vi "H5Pget_alloc_time.vi"(6 "error in (no error)":errorcluster, 9 "HDF5 Property Ref":T2) -> (0 "error out":errorcluster, 2 "Alloc Time":T1 items=["H5D_ALLOC_TIME_ERROR"=-1, "H5D_ALLOC_TIME_DEFAULT"=0, "H5D_ALLOC_TIME_EARLY"=1, "H5D_ALLOC_TIME_LATE"=2, "H5D_ALLOC_TIME_INCR"=3], 3 "HDF5 Ref out":T2)   [LabVIEW 2017]
doc: "Retrieves the timing for storage space allocation."
uses:
  <vilib>/UPVI/lvhdf5/library.llb/HDF5 Ref.ctl
  <vilib>/UPVI/lvhdf5/property.llb/H5D_alloc_time_t.ctl
  <vilib>/UPVI/lvhdf5/hdf5.dll
panel:
  # "LVHDF5 Toolkit\nCopyright (c) 2005-2013 by Jason D. Sommerville\nCopyright (c) 2014 by UPVI, LLC.\n\nThis use and distribution of this file is governed by the terms found in \nLICENSE.txt distributed with this toolkit and installed at\n <user.lib>\\_lvhdf5\\LICENSE.txt"
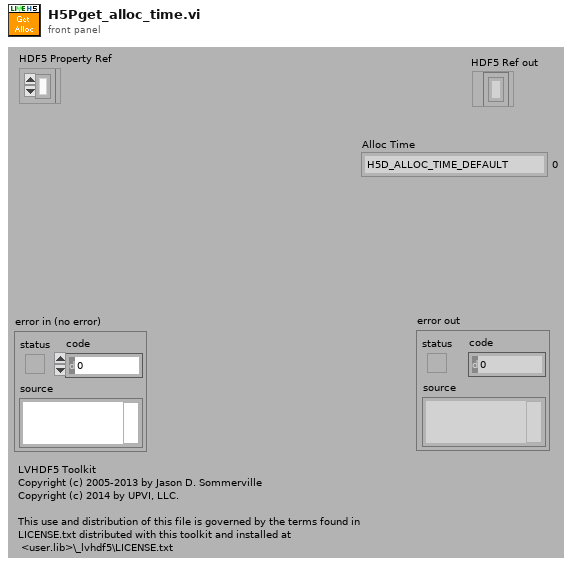
[diagram p1: front panel]
types:
  T1 = typedef "H5D_alloc_time_t.ctl" = i32
  T2 = typedef "HDF5 Ref.ctl" = refnum<k1>
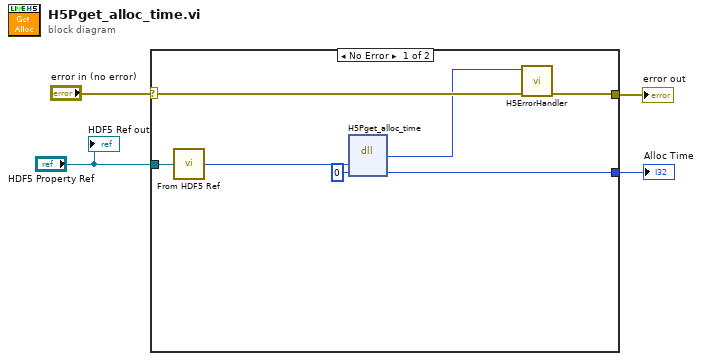
[diagram p0: block diagram]
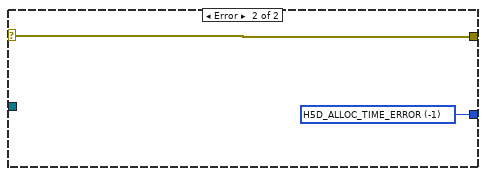
[diagram p2: hidden frame]
diagram:
  n1 = case shown="No Error" "error in (no error)" {
    selector: "error in (no error)" -> [w11 w13]
    tunnel: [w10 w13] -> w3
    tunnel: "HDF5 Property Ref" -> [w9 _]
    tunnel: [w5 w12] -> w1
    frame No Error {
      n2 = call <vilib>:"From HDF5 Ref.vi"("HDF5 Ref"=w9) -> ("I32"=w8:i32)
      n3 = dll-call lib="C:/Program Files/National Instruments/LabVIEW 2017/vi.lib/UPVI/lvhdf5/hdf5.dll" fn="H5Pget_alloc_time"("plist_id"=w8, "alloc_time"=0 ("fill_time")) -> (w7:i32, "alloc_time"=w5:i32)  [unwired: 4 in, 2 out]
      n4 = call <vilib>:"H5ErrorHandler.vi"("error in (no error)"=w11, "herr_t"=w7) -> ("error out"=w10:errorcluster)  [unwired: 3 in, 4 out]
    }
    frame Error {
      w12 = T1 -1 items=["H5D_ALLOC_TIME_ERROR"=-1, "H5D_ALLOC_TIME_DEFAULT"=0, "H5D_ALLOC_TIME_EARLY"=1, "H5D_ALLOC_TIME_LATE"=2, "H5D_ALLOC_TIME_INCR"=3] ("Alloc Time")
    }
  }
  "error out" <- w3
  "Alloc Time" <- w1
  "HDF5 Ref out" <- "HDF5 Property Ref"
